vi "Field Draw Robot.vi"(0 "Offset":T17, 1 "picture in":picture, 3 "Draw Number":bool, 5 "Detection Robot":T15 {"height" format="%+4.3f"; "pixel_y" format="%+4.3f"; "pixel_x" format="%+4.3f"; "orientation" format="%+4.3f"; "y" format="%+4.3f"; "confidence" format="%4.3f"; "x" format="%+4.3f"}, 9 "Scale mm/pixel":sgl, 11 "color(black)":u32(colorbox)=16775978, 12 "Robot":T2={"id"=0, "function"=enum."Attacker", "x"=0.0, "y"=0.0, "orientation"=0.0, "v_tangent"=0.0, "v_normal"=0.0, "v_ang"=0.0, "kick_x"=0.0, "kick_z"=0.0, "dribble"=FALSE, "Timestamp"=timestamp(0 s since 1904-01-01), "estimatives"={"est_v_tangent"=0.0, "est_v_normal"=0.0, "est_vx"=0.0, "est_vy"=0.0, "Pos Robot Est"=[]}, "dest_x_kick"=0.0, "dest_y_kick"=0.0, "Gap Coord"=[], "States"=enum."GoToTangent", "Path "=[], "Path  Smooth"=[], "Dest"=[]}, 13 "IA state":T1={"our_robots"=[], "enemy_robots"=[], "balls"=[], "geometry"={"line_width"=0, "field_length"=0, "field_width"=0, "boundary_width"=0, "referee_width"=0, "goal_width"=0, "goal_depth"=0, "goal_wall_width"=0, "center_circle_radius"=0, "defense_radius"=0, "defense_stretch"=0, "free_kick_from_defense_dist"=0, "penalty_spot_from_field_line_dist"=0, "penalty_line_from_spot_dist"=0}, "IA Judge"={"stage"="", "command"="", "our_goalie_id"=0.0, "enemy_goalie_id"=0.0, "command enum"=enum."Halt", "Time"=enum."Azul"}, "Received Timestamp"=timestamp(0 s since 1904-01-01), "Events"={"Touch"=FALSE, "Ball out"=FALSE, "id touch"=0.0, "Ball out of \nVision"=FALSE, "Ball inside \nGoalie area"=FALSE, "Robot not responding"=FALSE, "Robots responding status"=[1.0, 1.0, 1.0, 1.0, 1.0, 1.0], "Enemy Ball \nPossession"=FALSE, "Pass State"=FALSE, "id end of pass"=0.0, "Kick"=FALSE, "Id ini Possession"=0.0, "Ball Possesion"=FALSE, "Id Possesion"=0.0, "Direct Kick"=FALSE, "2nd Strk Ativo"=FALSE}}, 14 "IA Judge.Time":enum16{"Azul", "Amarelo"}(ring), 15 "Draw Targets?":T12) -> (4 "picture out":picture)   [LabVIEW 2018]
uses:
  <vilib>/Utility/miscctls.llb/LVBoundsTypeDef.ctl
  SSL Detection Robot.ctl
  <vilib>/Analysis/Matrix/Datatypes/RealMatrix.ctl
  Core/AI Robot.ctl
  Intel/Functions Enum.ctl
  Intel/AttackerStates.ctl
  Path Planning/RRT/PathDests.ctl
  Path Planning/RRT/PathDest.ctl
  DrawTargets.ctl
  Core/AI Input.ctl
  Core/AI Ball.ctl
  Core/Field Size.ctl
  Core/AI Judge.ctl
  Intel/Command Enum.ctl
  Util/Events/Events.ctl
  <vilib>/Analysis/coordinate.llb/2D Cartesian Coordinate Rotation (Scalar).vi
  <vilib>/Analysis/NI_AALPro.lvlib
  <vilib>/Analysis/Matrix/NI_Matrix.lvlib
panel:
  in  "pen Chute":T13={"Width"=3, "Style"=enum."Solid"}
  in  "pen":T14={"Width"=1.0, "Style"=enum."Solid"}
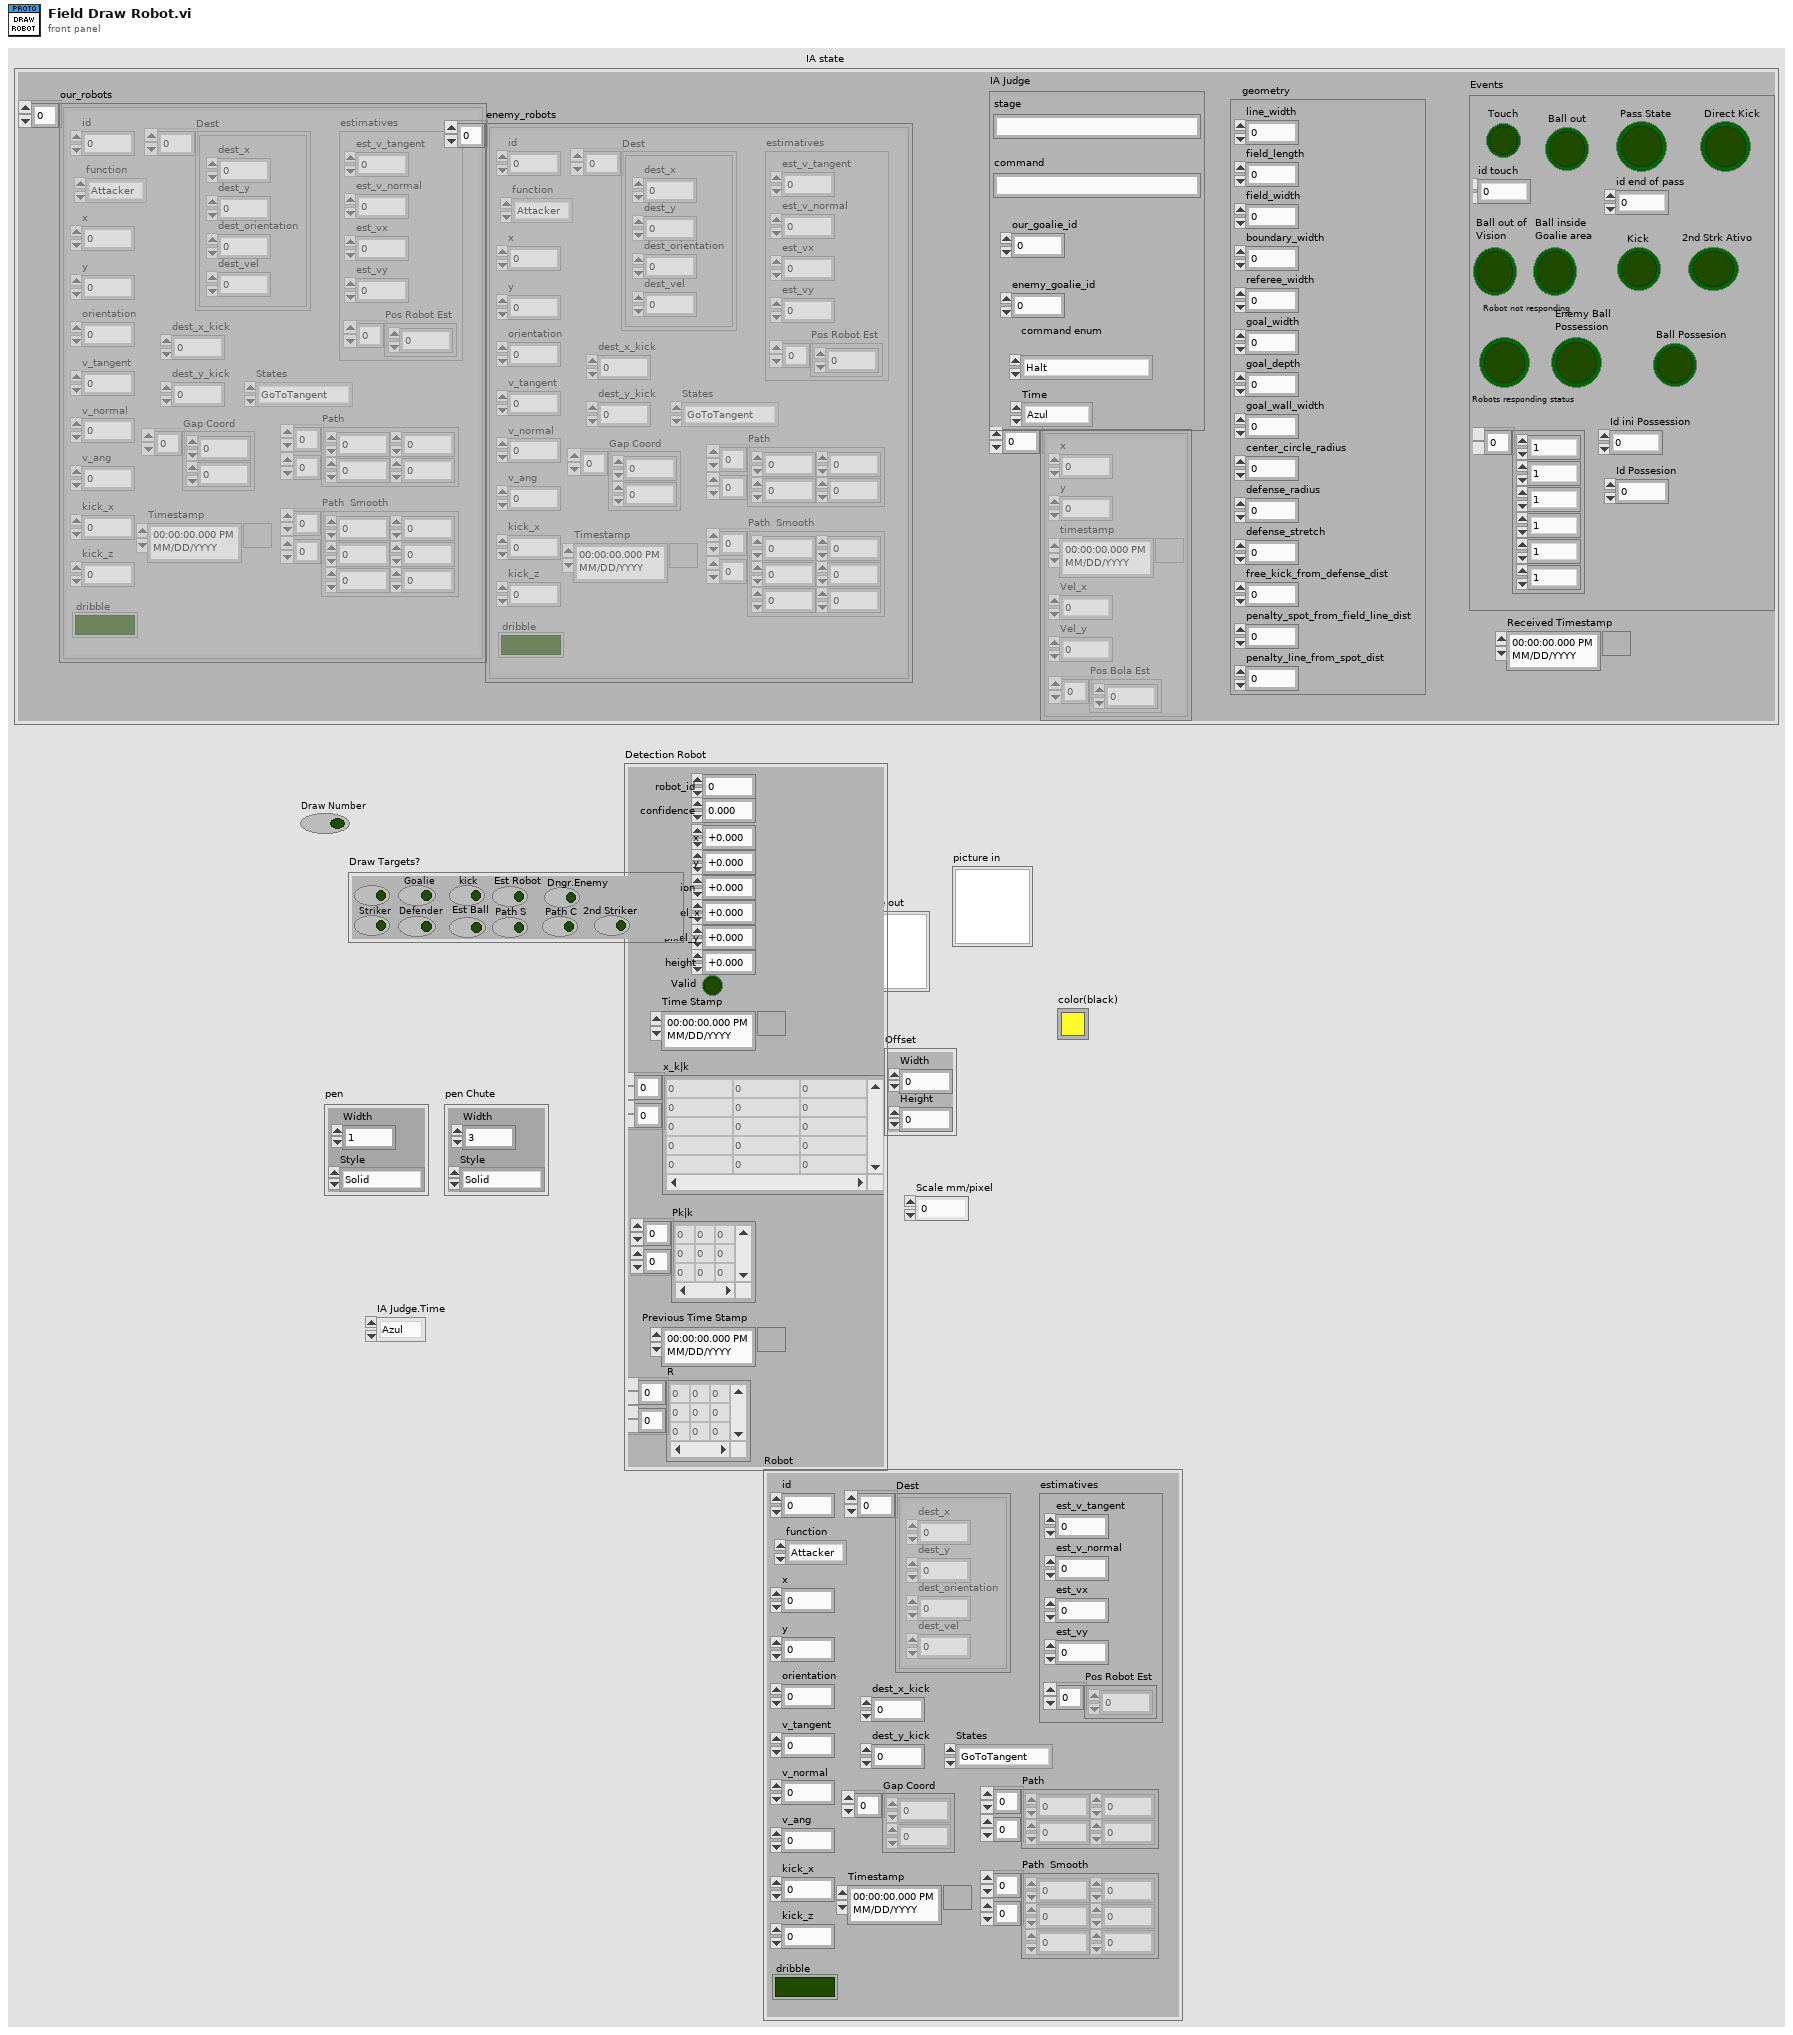
[diagram p1: front panel]
types:
  T1 = typedef "AI Input.ctl" = cluster{"our_robots":T2[], "enemy_robots":T2[], "balls":T7[], "geometry":T8, "IA Judge":T9, "Received Timestamp":timestamp, "Events":T11}
  T2 = typedef "AI Robot.ctl" = cluster{"id":u32, "function":T3, "x":dbl, "y":dbl, "orientation":dbl, "v_tangent":dbl, "v_normal":dbl, "v_ang":dbl, "kick_x":dbl, "kick_z":dbl, "dribble":bool, "Timestamp":timestamp, "estimatives":cluster{"est_v_tangent":dbl, "est_v_normal":dbl, "est_vx":dbl, "est_vy":dbl, "Pos Robot Est":dbl[]}, "dest_x_kick":dbl, "dest_y_kick":dbl, "Gap Coord":dbl[], "States":T4, "Path ":dbl[][], "Path  Smooth":dbl[][], "Dest":T5}
  T3 = typedef "Functions Enum.ctl" = enum16{"2nd Striker", "Attacker", "Goalie", "Defender", "Striker", "Goto 0", "Dummy", "Kicker", "ZigZag 0", "ZigZag 1", "ZigZag 2", "ZigZag 3", "ZigZag 4", "ZigZag 5", "ZigZag 6", "ZigZag 7", "ZigZag 8", ""}
  T4 = typedef "AttackerStates.ctl" = enum16{"Pass", "GoToTangent", "BallGetting", "GoToKick", ""}
  T5 = typedef "PathDests.ctl" = T6[]
  T6 = typedef "PathDest.ctl" = cluster{"dest_x":dbl, "dest_y":dbl, "dest_orientation":dbl, "dest_vel":dbl}
  T7 = typedef "AI Ball.ctl" = cluster{"x":dbl, "y":dbl, "timestamp":timestamp, "Vel_x":dbl, "Vel_y":dbl, "Pos Bola Est":dbl[]}
  T8 = typedef "Field Size.ctl" = cluster{"line_width":u32, "field_length":u32, "field_width":u32, "boundary_width":u32, "referee_width":u32, "goal_width":u32, "goal_depth":u32, "goal_wall_width":u32, "center_circle_radius":u32, "defense_radius":u32, "defense_stretch":u32, "free_kick_from_defense_dist":u32, "penalty_spot_from_field_line_dist":u32, "penalty_line_from_spot_dist":u32}
  T9 = typedef "AI Judge.ctl" = cluster{"stage":string, "command":string, "our_goalie_id":dbl, "enemy_goalie_id":dbl, "command enum":T10, "Time":enum16{"Azul", "Amarelo"}}
  T10 = typedef "Command Enum.ctl" = enum16{"Halt", "Stop", "Force Start", "PKA Normal Start", "Prepare Kickoff Ally", "PKE Normal Start", "Prepare Kickoff Enemy", "Prepare Penalty Ally", "PPA Normal Start", "Prepare Penalty Enemy", "PPE Normal Start", "Direct Free Enemy", "Direct Free Ally", "Indirect Free Enemy", "Indirect Free Ally", "Timeout Enemy", "Timeout Ally", "Goal Enemy", "Goal Ally", "Ball Placement Enemy", "Ball Placement Ally", "Normal Half Time", "Extra Time Break", "Extra Half Time", "None", "Post Game"}
  T11 = typedef "Events.ctl" = cluster{"Touch":bool, "Ball out":bool, "id touch":dbl, "Ball out of \nVision":bool, "Ball inside \nGoalie area":bool, "Robot not responding":bool, "Robots responding status":dbl[], "Enemy Ball \nPossession":bool, "Pass State":bool, "id end of pass":dbl, "Kick":bool, "Id ini Possession":dbl, "Ball Possesion":bool, "Id Possesion":dbl, "Direct Kick":bool, "2nd Strk Ativo":bool}
  T12 = typedef "DrawTargets.ctl" = cluster{"Attacker":bool, "Striker":bool, "Goalie":bool, "Defender":bool, "kick":bool, "Est Ball":bool, "Est Robot":bool, "Path S":bool, "Path C":bool, "Dngr.Enemy":bool, "2nd Striker":bool}
  T13 = cluster{"Width":u16, "Style":enum32{"Solid", "Dash", "Dot", "DashDot", "DashDotDot"}}
  T14 = cluster{"Width":dbl, "Style":enum32{"Solid", "Dash", "Dot", "DashDot", "DashDotDot"}}
  T15 = typedef "SSL Detection Robot.ctl" = cluster{"x":sgl, "robot_id":u32, "confidence":sgl, "y":sgl, "orientation":sgl, "pixel_x":sgl, "pixel_y":sgl, "height":sgl, "Valid":bool, "Time Stamp":timestamp, "x_k|k":T16, "Pk|k":T16, "Previous Time Stamp":timestamp, "R":T16}
  T16 = typedef "NI_Matrix.lvlib/RealMatrix.ctl" = dbl[][]
  T17 = typedef "LVBoundsTypeDef.ctl" = cluster{"Width":u32, "Height":u32}
  T18 = cluster{"horizontal":enum16{"left", "center", "right"}, "vertical":enum16{"top", "center", "bottom"}}
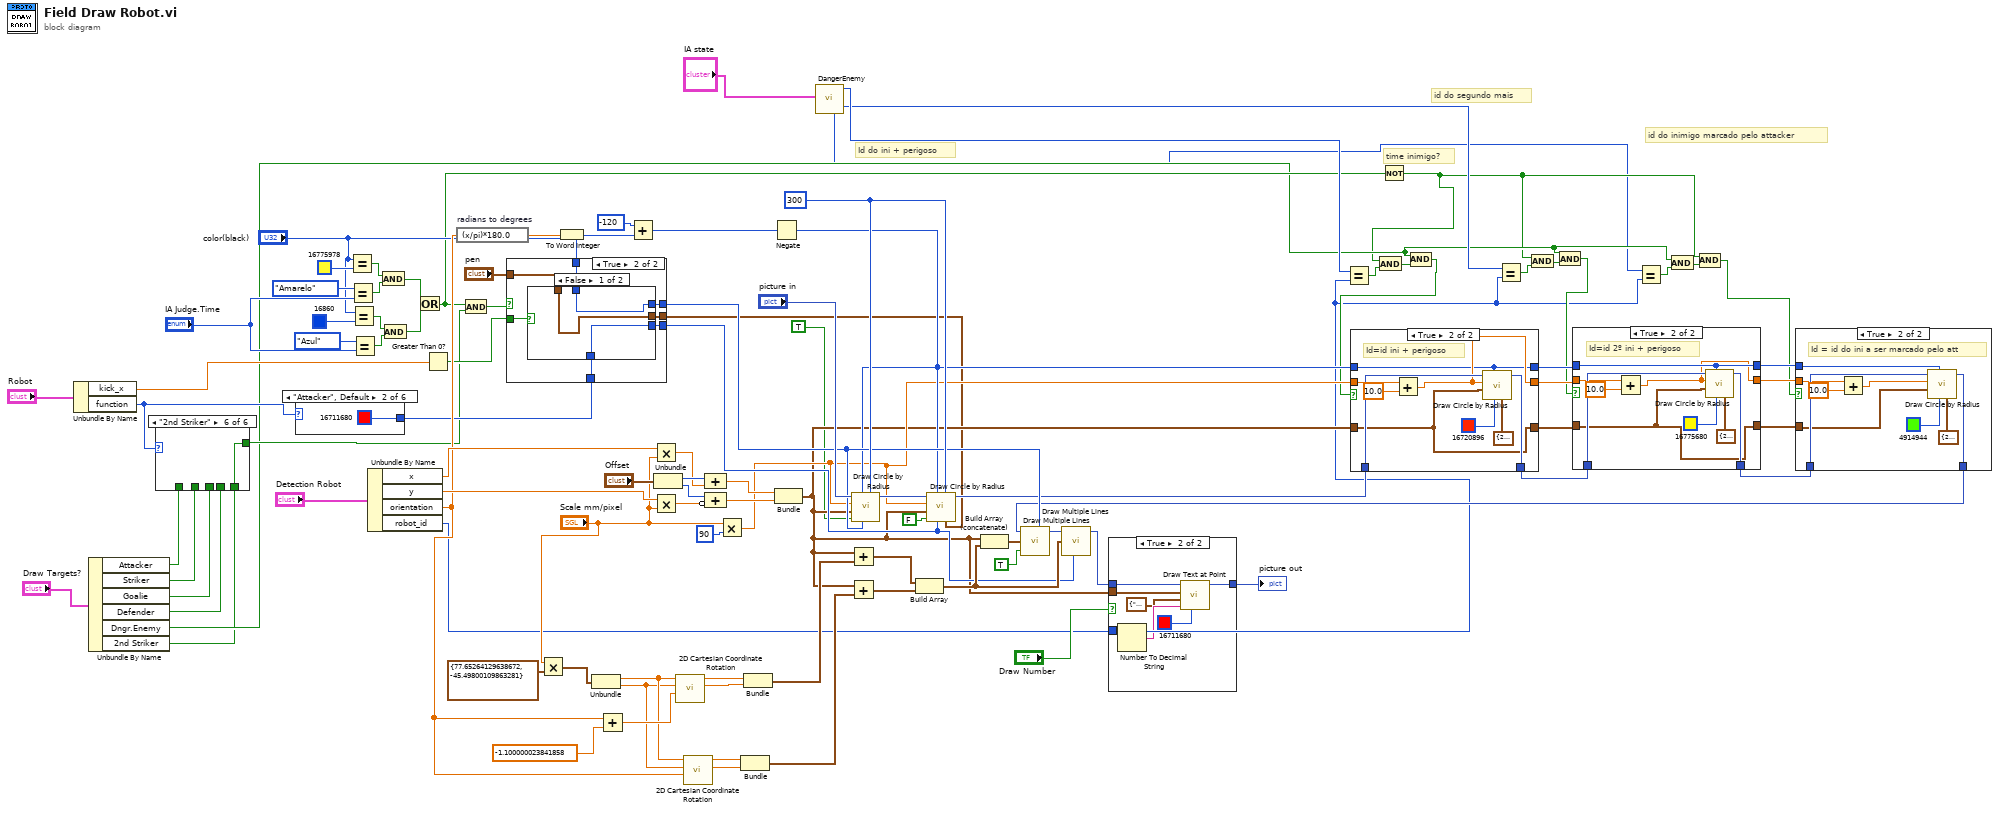
[diagram p0: block diagram]
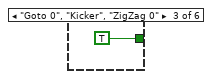
[diagram p7: hidden frame]
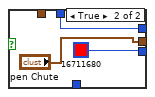
[diagram p11: hidden frame]
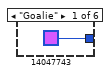
[diagram p12: hidden frame]
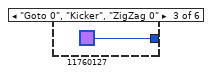
[diagram p13: hidden frame]
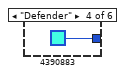
[diagram p14: hidden frame]
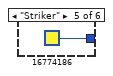
[diagram p15: hidden frame]
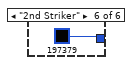
[diagram p16: hidden frame]
diagram:
  w86 = i16 300 ("arc size(360)")
  # "id do inimigo marcado pelo attacker"
  # "id do segundo mais"
  # "time inimigo?"
  # "Id do ini + perigoso"
  n1 = Unbundle By Name("Robot") -> ("kick_x"=w60:dbl, "function"=w36:T3)
  n2 = Unbundle By Name("Draw Targets?") -> ("Attacker"=w42:bool, "Striker"=w41:bool, "Goalie"=w40:bool, "Defender"=w39:bool, "Dngr.Enemy"=w5:bool, "2nd Striker"=w1:bool)
  n3 = case shown="\"2nd Striker\"" w36 {
    tunnel: [w103 w104 TRUE ("Draw Target Striker?") w106 w107 w108] -> w37
    tunnel: w39 -> [_ _ _ w106 _ _]
    tunnel: w41 -> [_ _ _ _ w107 _]
    tunnel: w42 -> [w103 _ _ _ _ _]
    tunnel: w40 -> [_ w104 _ _ _ _]
    tunnel: w1 -> [_ _ _ _ _ w108]
    frame "Attacker", Default {
    }
    frame "Goalie" {
    }
    frame "Goto 0", "Kicker", "ZigZag 0" {
    }
    frame "Defender" {
    }
    frame "Striker" {
    }
    frame "2nd Striker" {
    }
  }
  n4 = case shown="\"Attacker\", Default" w36 {
    tunnel: [u32 14047743 ("color(black)") u32 16711680 ("color(black)") u32 11760127 ("color(black)") u32 4390883 ("color(black)") u32 16774186 ("color(black)") u32 197379 ("color(black)")] -> w46
    frame "Goalie" {
    }
    frame "Attacker", Default {
    }
    frame "Goto 0", "Kicker", "ZigZag 0" {
    }
    frame "Defender" {
    }
    frame "Striker" {
    }
    frame "2nd Striker" {
    }
  }
  n5 = Equal?(x="color(black)", y=u32 16775978 ("color(black)")) -> (x = y?=w53:bool)
  n6 = Equal?(x=enum16{"Azul", "Amarelo"}."Amarelo", y="IA Judge.Time") -> (x = y?=w54:bool)
  n7 = Equal?(x="color(black)", y=u32 16860 ("color(black)")) -> (x = y?=w50:bool)
  n8 = Equal?(x=enum16{"Azul", "Amarelo"}."Azul", y="IA Judge.Time") -> (x = y?=w51:bool)
  n9 = Unbundle By Name("Detection Robot") -> ("x"=w100:sgl, "y"=w101:sgl, "orientation"=w72:sgl, "robot_id"=w6:u32)
  n10 = And(x=w53, y=w54) -> (x .and. y?=w48:bool)
  n11 = And(x=w50, y=w51) -> (x .and. y?=w47:bool)
  n12 = Or(x=w48, y=w47) -> (x .or. y?=w17:bool)
  n13 = Greater Than 0?(x=w60) -> (x > 0?=w45:bool)
  n14 = expression code="(x/pi)*180.0" "radians to degrees"(w72) -> (w90:sgl)
  n15 = And(x=w17, y=w37) -> (x .and. y?=w38:bool)
  n16 = case shown="True" w38 {
    tunnel: [w116 w123] -> w58
    tunnel: [w116 w122] -> w57
    tunnel: "color(black)" -> [w116 w121]
    tunnel: w46 -> [_ w120]
    tunnel: [w115 w119] -> w30
    tunnel: w45 -> [_ w118]
    tunnel: "pen" -> [w115 w117]
    frame False {
    }
    frame True {
      n17 = case shown="False" w118 {
        tunnel: [w125 u32 16711680 ("color(black)")] -> w122
        tunnel: w121 -> [w126 w128]
        tunnel: [w126 w128] -> w123
        tunnel: w120 -> [w125 _]
        tunnel: [w124 "pen Chute"] -> w119
        tunnel: w117 -> [w124 _]
        frame False {
        }
        frame True {
        }
      }
    }
  }
  n18 = Multiply(x="Scale mm/pixel", y=cluster{sgl, sgl} {77.65264, -45.498} ("appended array")) -> (x*y=w67:cluster{sgl, sgl})
  n19 = To Word Integer(number=w90) -> (16bit integer=w89:i16)
  n20 = Unbundle(w67) -> (w74:sgl, w73:sgl)
  n21 = Add(x=w72, y=sgl -1.1 ("theta")) -> (x+y=w75:sgl)
  n22 = Add(x=i16 -120, y=w89) -> (x+y=w88:i16)
  n23 = Multiply(x=w100, y="Scale mm/pixel") -> (x*y=w96:sgl)
  n24 = Multiply(x=w101, y="Scale mm/pixel") -> (x*y=w93:sgl)
  n25 = Unbundle("Offset") -> ("Width"=w97:u32, "Height"=w94:u32)
  n26 = call-poly <vilib>:"2D Cartesian Coordinate Rotation.vi"("theta"=w75, "y"=w73, "x"=w74) -> ("y out"=w77:dbl, "x out"=w78:dbl)  [unwired: 6 in, 1 out]
  n27 = call-poly <vilib>:"2D Cartesian Coordinate Rotation.vi"("theta"=w72, "y"=w73, "x"=w74) -> ("y out"=w70:dbl, "x out"=w71:dbl)  [unwired: 6 in, 1 out]
  n28 = Compound Arithmetic op=ADD(w97, w96) -> (w95:sgl)
  n29 = Compound Arithmetic op=ADD(w94, invert w93) -> (w92:sgl)
  n30 = Multiply(x="Scale mm/pixel", y=i16 90 ("radius")) -> (x*y=w33:sgl)
  n31 = Bundle("x out"=w71, "y out"=w70) -> (w66:cluster{"x out":dbl, "y out":dbl})  [unwired: 1 in]
  n32 = Bundle("x out"=w78, "y out"=w77) -> (w65:cluster{"x out":dbl, "y out":dbl})  [unwired: 1 in]
  n33 = Negate(x=w88) -> (-x=w35:i16)
  n34 = Bundle(w95, w92) -> (w32:cluster{sgl, sgl})  [unwired: 1 in]
  n35 = call "DangerEnemy.vi"("IA Input"="IA state") -> ("id do segundo inimigo\nmais perigoso"=w23:i32, "id do inimigo\nmais perigoso"=w25:u32, "Id do Inimigo Mais Próximo"=w2:u32)  [unwired: 5 in, 3 out]
  n36 = Add(x=w32, y=w65) -> (x+y=w63:cluster{dbl, dbl})
  n37 = Add(x=w32, y=w66) -> (x+y=w64:cluster{dbl, dbl})
  n38 = call <vilib>:"Draw Circle by Radius.vi"("arc size(360)"=w86, "color(black)"=w58, "start angle(0)"=w35, "fill?(F)"=TRUE, "pixel center"=w32, "radius"=w33, "picture"="picture in") -> ("new picture"=w61:picture)  [unwired: 4 in]
  n39 = Build Array(w63, w64) -> (w83:cluster{dbl, dbl}[])
  n40 = call <vilib>:"Draw Circle by Radius.vi"("pen"=w30, "arc size(360)"=w86, "color(black)"=w57, "start angle(0)"=w35, "fill?(F)"=FALSE, "pixel center"=w32, "radius"=w33, "picture"=w61) -> ("new picture"=w34:picture)  [unwired: 3 in]
  n41 = Build Array (concatenate)(w32, w83) -> (w81:cluster{dbl, dbl}[])
  n42 = Equal?(x=w25, y=w6) -> (x = y?=w28:bool)
  n43 = Not(x=w17) -> (.not. x?=w4:bool)
  n44 = And(x=w4, y=w28) -> (x .and. y?=w18:bool)
  n45 = And(x=w5, y=w18) -> (x .and. y?=w16:bool)
  n46 = case shown="True" w16 {
    tunnel: w35 -> [w132 w135]
    tunnel: w34 -> [w133 w142]
    tunnel: [w133 w141] -> w22
    tunnel: w33 -> [w131 w140]
    tunnel: w32 -> [w130 w134]
    tunnel: [w132 w135] -> w21
    tunnel: [w131 w136] -> w20
    tunnel: [w130 w134] -> w19
    frame False {
    }
    frame True {
      # "Id=id ini + perigoso"
      n47 = Add(x=w140, y=sgl 10.0) -> (x+y=w136:sgl)
      n48 = call <vilib>:"Draw Circle by Radius.vi"("pen"=T13 {"Width"=2, "Style"=enum."Solid"}, "color(black)"=u32 16720896, "start angle(0)"=w135, "pixel center"=w134, "radius"=w136, "picture"=w142) -> ("new picture"=w141:picture)  [unwired: 5 in]
    }
  }
  n49 = Equal?(x=w23, y=w6) -> (x = y?=w24:bool)
  n50 = And(x=w4, y=w24) -> (x .and. y?=w15:bool)
  n51 = And(x=w5, y=w15) -> (x .and. y?=w14:bool)
  n52 = case shown="True" w14 {
    tunnel: w21 -> [w145 w149]
    tunnel: w22 -> [w146 w155]
    tunnel: [w146 w154] -> w10
    tunnel: w20 -> [w144 w153]
    tunnel: w19 -> [w143 w147]
    tunnel: [w145 w149] -> w13
    tunnel: [w144 w148] -> w12
    tunnel: [w143 w147] -> w11
    frame False {
    }
    frame True {
      # "Id=id 2º ini + perigoso"
      n53 = Add(x=w153, y=sgl 10.0) -> (x+y=w148:sgl)
      n54 = call <vilib>:"Draw Circle by Radius.vi"("pen"=T13 {"Width"=2, "Style"=enum."Solid"}, "color(black)"=u32 16775680, "start angle(0)"=w149, "pixel center"=w147, "radius"=w148, "picture"=w155) -> ("new picture"=w154:picture)  [unwired: 5 in]
    }
  }
  n55 = Equal?(x=w2, y=w6) -> (x = y?=w7:bool)
  n56 = And(x=w5, y=w7) -> (x .and. y?=w8:bool)
  n57 = And(x=w4, y=w8) -> (x .and. y?=w3:bool)
  n58 = case shown="True" w3 {
    tunnel: w13 -> [_ w165]
    tunnel: w10 -> [w156 w164]
    tunnel: [w156 w163] -> w9
    tunnel: w12 -> [_ w162]
    tunnel: w11 -> [_ w161]
    frame False {
    }
    frame True {
      # "Id = id do ini a ser marcado pelo att"
      n59 = Add(x=w162, y=sgl 10.0) -> (x+y=w160:sgl)
      n60 = call <vilib>:"Draw Circle by Radius.vi"("pen"=T13 {"Width"=2, "Style"=enum."Solid"}, "color(black)"=u32 4914944, "start angle(0)"=w165, "pixel center"=w161, "radius"=w160, "picture"=w164) -> ("new picture"=w163:picture)  [unwired: 5 in]
    }
  }
  n61 = call <vilib>:"Draw Multiple Lines.vi"("picture"=w9, "line endpoints"=w81, "fill?(F)"=TRUE, "color(black)"=w58) -> ("new picture"=w82:picture)  [unwired: 5 in]
  n62 = call <vilib>:"Draw Multiple Lines.vi"("picture"=w82, "line endpoints"=w83, "color(black)"=w57) -> ("new picture"=w84:picture)  [unwired: 6 in]
  n63 = case shown="True" "Draw Number" {
    tunnel: [w166 w173] -> w87
    tunnel: w6 -> [_ w171]
    tunnel: w84 -> [w166 w169]
    tunnel: w32 -> [_ w168]
    frame False {
    }
    frame True {
      n64 = Number To Decimal String(number=w171) -> (decimal integer string=w172:string)  [unwired: 1 in]
      n65 = call <vilib>:"Draw Text at Point.vi"("text color(black)"=u32 16711680, "text"=w172, "alignment(left, top)"=T18 {"horizontal"=enum."center", "vertical"=enum."center"}, "origin"=w168, "picture"=w169) -> ("new picture"=w173:picture)  [unwired: 5 in, 1 out]
    }
  }
  "picture out" <- w87
